vi "DoNotSetChannelList.vi"() -> (3 "DoNotSetChannels[]":string[](array[string]))   [LabVIEW 2020]
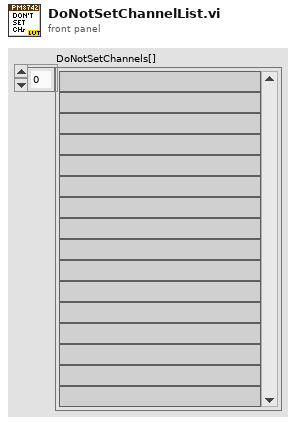
[diagram p1: front panel]
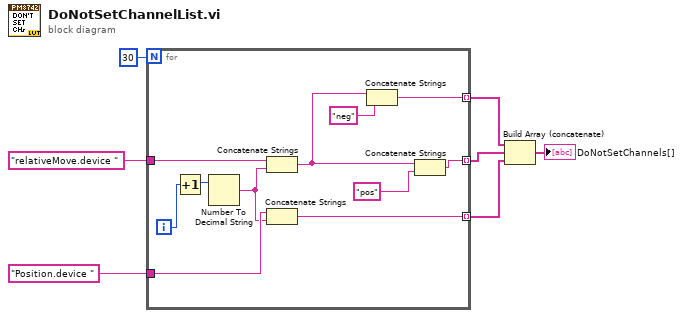
[diagram p0: block diagram]
diagram:
  n1 = for {
    N: 30 -> [_]
    tunnel: "relativeMove.device " -> [w16]
    tunnel: [w13] -> w5 mode=indexing
    tunnel: [w12] -> w6 mode=indexing
    tunnel: "Position.device " -> [w11]
    tunnel: [w9] -> w7 mode=indexing
    i -> [w17]
    n2 = Increment(x=w17) -> (x+1=w18:i32)
    n3 = Number To Decimal String(number=w18) -> (decimal integer string=w10:string)  [unwired: 1 in]
    n4 = Concatenate Strings(w16, w10) -> (w8:string)
    n5 = Concatenate Strings(w11, w10) -> (w9:string)
    n6 = Concatenate Strings(w8, "neg") -> (w13:string)
    n7 = Concatenate Strings(w8, "pos") -> (w12:string)
  }
  n8 = Build Array (concatenate)(w5, w6, w7) -> (→"DoNotSetChannels[]":string[])
